vi "function1.vi"(9 "b":dbl, 10 "x":dbl, 11 "a":dbl) -> (3 "y=a*x*+b":dbl)   [LabVIEW 2019]
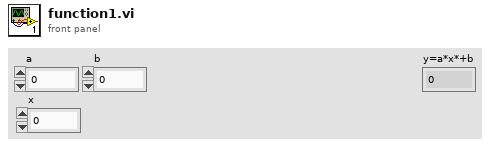
[diagram p1: front panel]
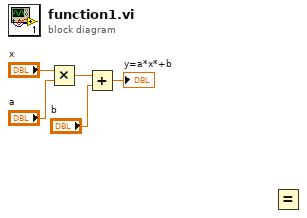
[diagram p0: block diagram]
diagram:
  n1 = Multiply(x="x", y="a") -> (x*y=w5:dbl)
  n2 = Add(x=w5, y="b") -> (x+y=→"y=a*x*+b":dbl)
  n3 = Equal?() -> ()  [unwired: 2 in, 1 out]
